vi "Helmholtz2D_Check Input_RHS.vi"(8 "error in (no error)":errorcluster, 10 "Domain":T1={"x"={"start x"=0.0, "end x"=1.0, "# of x-points"=11}, "y"={"start y"=0.0, "end y"=1.0, "# of y-points"=11}}, 11 "F(x, y)":dbl[][](array[numeric])) -> (0 "error out":errorcluster)   [LabVIEW 2020, in "NI_PDE.lvlib"]
uses:
  <vilib>/gmath/NI_PDE.lvlib
  <vilib>/gmath/pde.llb/Common/PDE_Error.ctl
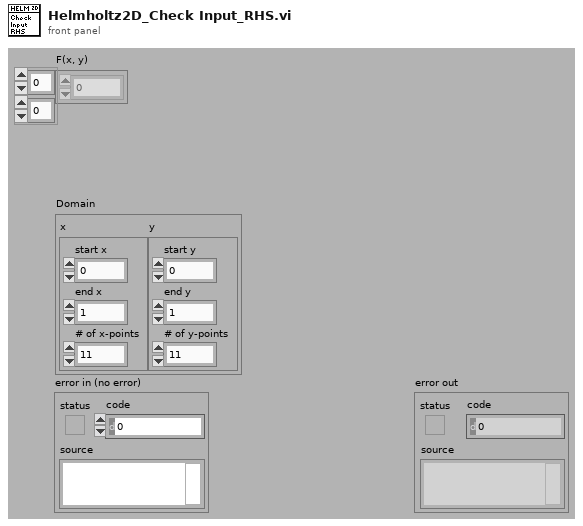
[diagram p1: front panel]
types:
  T1 = cluster{"x":cluster{"start x":dbl, "end x":dbl, "# of x-points":i32}, "y":cluster{"start y":dbl, "end y":dbl, "# of y-points":i32}}
  T2 = typedef "NI_PDE.lvlib/PDE_Error.ctl" = enum16{"No Error", "k is zero", "End point <= start point", "# of time steps < 2", "# of spatial points < 3", "# of grid < 1 for FEM", "# of boundary < 3 for FEM", "Incompatible RHS size", "Incompatible BC size", "Incompatible IC size", "PDE class conflict", "RHS class conflict", "Domain class conflict", "BC class conflict", "IC class conflict"}
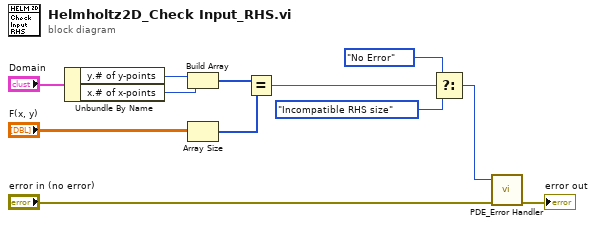
[diagram p0: block diagram]
diagram:
  n1 = Unbundle By Name("Domain") -> ("y.# of y-points"=w7:i32, "x.# of x-points"=w5:i32)
  n2 = Build Array(w7, w5) -> (w6:i32[])
  n3 = Array Size(array="F(x, y)") -> (size(s)=w8:i32[])
  n4 = Equal?(x=w6, y=w8) -> (x = y?=w4:bool)
  n5 = Select(t=PDE_Error."No Error" ("PDE error"), s=w4, f=PDE_Error."Incompatible RHS size" ("PDE error")) -> (s? t:f=w3:T2)
  n6 = call <vilib>:"PDE_Error Handler.vi"("error in (no error)"="error in (no error)", "PDE error"=w3) -> ("error out"=→"error out":errorcluster)  [unwired: 9 out]
